vi "test_LoadCommandlineArgs_AddPackedLibWithAllParameters.vi"() -> (3 "Pass?":bool)   [LabVIEW 2019, in "Tests.SolutionBuilder.lvlib"]
uses:
  Tests.SolutionBuilder.lvlib
  SolutionBuilder/Community/Options.ctl
  SolutionBuilder/ProjectItem/ProjectItem.lvclass/ProjectItem.ctl
  SolutionBuilder/SolutionBuilder.lvclass
  SolutionBuilder/ProjectItem/ProjectItem.lvclass
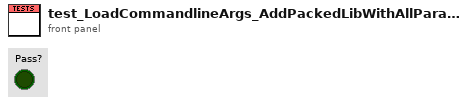
[diagram p1: front panel]
types:
  T1 = typedef "SolutionBuilder.lvlib/SolutionBuilder.lvclass/Options.ctl" = cluster{"Path":path, "Preview?":bool, "Quiet?":bool, "Log file":path, "Success file":path, "Rebuild?":bool, "Keep split projects?":bool}
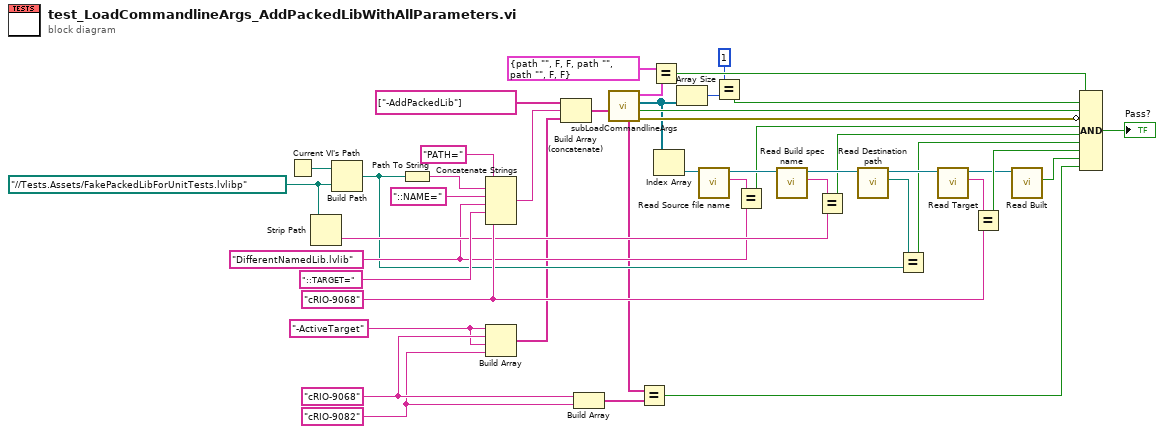
[diagram p0: block diagram]
diagram:
  w3 = "cRIO-9082"
  w7 = "cRIO-9068"
  w4 = "-ActiveTarget"
  w43 = "cRIO-9068" ("string")
  w34 = "DifferentNamedLib.lvlib" ("string")
  w37 = path "../../Tests.Assets/FakePackedLibForUnitTests.lvlibp" ("Path")
  n1 = Current VI's Path() -> (path=w20:path)
  n2 = Strip Path(path=w37) -> (name=w38:string)  [unwired: 1 out]
  n3 = Build Path(base path=w20, name or relative path=w37) -> (appended path=w30:path)
  n4 = Path To String(path=w30) -> (string=w32:string)
  n5 = Concatenate Strings("PATH=" ("string"), w32, "::NAME=" ("string"), w34, "::TARGET=" ("string"), w43) -> (w33:string)
  n6 = Build Array(w4, w7, w4, w3) -> (w8:string[])
  n7 = Build Array (concatenate)(string[] ["-AddPackedLib"] ("App.Args"), w33, w8) -> (w19:string[])
  n8 = Build Array(w7, w3) -> (w6:string[])
  n9 = call "subLoadCommandlineArgs.vi"("App.Args"=w19) -> ("error out"=w24:errorcluster, "From command line?"=w28:bool, "Pre-built libraries"=w18:refnum<class "ProjectItem.lvclass">[], "Options"=w26:T1, "Active targets"=w5:string[])  [unwired: 6 in]
  n10 = Equal?(x=w5, y=w6) -> (x = y?=w1:bool)
  n11 = Equal?(x=T1 {"Path"=path "", "Preview?"=FALSE, "Quiet?"=FALSE, "Log file"=path "", "Success file"=path "", "Rebuild?"=FALSE, "Keep split projects?"=FALSE} ("Options"), y=w26) -> (x = y?=w27:bool)
  n12 = Index Array(array=w18) -> (element=w17:refnum<class "ProjectItem.lvclass">)  [unwired: 1 in]
  n13 = Array Size(array=w18) -> (size(s)=w23:i32)
  n14 = call "Read Source file name.vi"("ProjectItem in"=w17) -> ("Source file name"=w14:string, "ProjectItem out"=w16:refnum<class "ProjectItem.lvclass">)  [unwired: 9 in]
  n15 = Equal?(x=1, y=w23) -> (x = y?=w21:bool)
  n16 = Equal?(x=w14, y=w34) -> (x = y?=w11:bool)
  n17 = call "Read Build spec name.vi"("ProjectItem in"=w16) -> ("Build spec name"=w13:string, "ProjectItem out"=w15:refnum<class "ProjectItem.lvclass">)  [unwired: 9 in]
  n18 = Equal?(x=w13, y=w38) -> (x = y?=w10:bool)
  n19 = call "Read Destination path.vi"("ProjectItem in"=w15) -> ("Destination path"=w12:path, "ProjectItem out"=w40:refnum<class "ProjectItem.lvclass">)  [unwired: 9 in]
  n20 = Equal?(x=w12, y=w30) -> (x = y?=w9:bool)
  n21 = call "Read Target.vi"("ProjectItem in"=w40) -> ("Target"=w42:string, "ProjectItem out"=w41:refnum<class "ProjectItem.lvclass">)  [unwired: 9 in]
  n22 = Equal?(x=w42, y=w43) -> (x = y?=w44:bool)
  n23 = call "Read Built.vi"("ProjectItem in"=w41) -> ("Built"=w2:bool)  [unwired: 9 in, 1 out]
  n24 = Compound Arithmetic op=AND(w27, w21, w28, invert w24, w11, w10, w9, w44, w2, w1) -> (→"Pass?":bool)
